vi "Evaluate Part 2.vi"() -> ()   [LabVIEW 2020]
uses:
  Stateless Network/Stateless Network.lvclass
panel:
  out "Steps":u64
  in  "Input":string
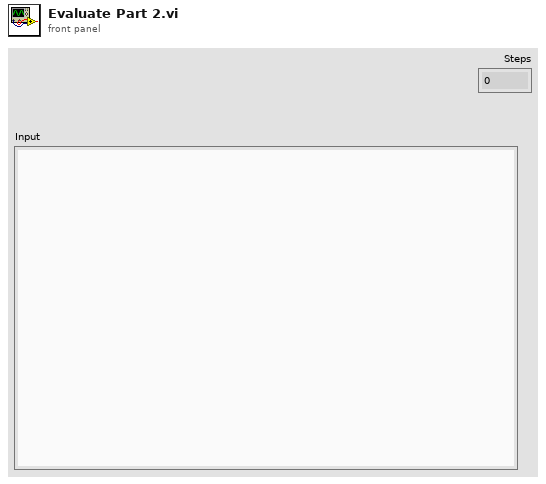
[diagram p1: front panel]
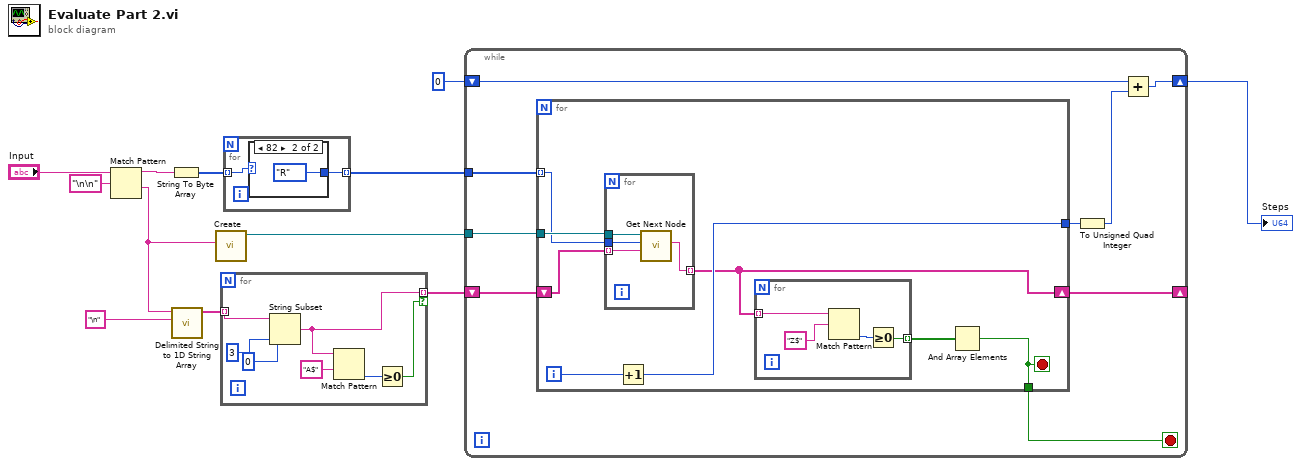
[diagram p0: block diagram]
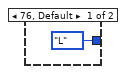
[diagram p2: hidden frame]
diagram:
  n1 = Match Pattern(string="Input", regular expression="\n\n" ("search string/char (-)")) -> (before substring=w10:string, after substring=w6:string)  [unwired: 1 in, 2 out]
  n2 = String To Byte Array(string=w10) -> (unsigned byte array=w9:u8[])
  n3 = call <vilib>:"Delimited String to 1D String Array.vi"("delimiter"="\n" ("search string/char (-)"), "delimited string"=w6) -> ("string array"=w2:string[])  [unwired: 9 in]
  n4 = call "Create.vi"("Input"=w6) -> ("Network"=w7:refnum<class "Stateless Network.lvclass">)  [unwired: 9 in, 1 out]
  n5 = for {
    tunnel: w2 -> [w14] mode=indexing
    tunnel: [w13] -> w1 mode=indexing if=w17
    n6 = String Subset(string=w14, offset (0)=0, length (rest)=3 ("length (rest)")) -> (substring=w13:string)
    n7 = Match Pattern(string=w13, regular expression="A$" ("y")) -> (offset past match=w18:i32)  [unwired: 1 in, 3 out]
    n8 = Greater Or Equal To 0?(x=w18) -> (x >= 0?=w17:bool)
  }
  n9 = for {
    tunnel: w9 -> [w21] mode=indexing
    tunnel: [w20] -> w8 mode=indexing
    n10 = case shown="82" w21 {
      tunnel: [enum16{"L", "R"}."L" ("Direction") enum16{"L", "R"}."R" ("Direction")] -> w20
      frame 76, Default {
      }
      frame 82 {
      }
    }
  }
  n11 = while {
    tunnel: w8 -> [w32]
    shift-right: [w27] -> _
    shift-left: w1 -> [w28]
    tunnel: w7 -> [w31]
    shift-right: [w25] -> w3
    shift-left: u64 0 -> [w26]
    stop <- w29 stop-if-true
    n12 = for {
      tunnel: w32 -> [w39] mode=indexing
      tunnel: [w37] -> w30
      tunnel: [w33] -> w29
      shift-right: [w35] -> w27
      shift-left: w28 -> [w36]
      tunnel: w31 -> [w40]
      i -> [w38]
      stop <- w33 stop-if-true
      n13 = for {
        tunnel: w39 -> [w47]
        tunnel: [w46] -> w35 mode=indexing
        tunnel: w36 -> [w45] mode=indexing
        tunnel: w40 -> [w48]
        n14 = call "Get Next Node.vi"("State"=w45, "Direction"=w47, "Network in"=w48) -> ("Node"=w46:string)  [unwired: 6 in, 2 out]
      }
      n15 = Increment(x=w38) -> (x+1=w37:i32)
      n16 = for {
        tunnel: w35 -> [w42] mode=indexing
        tunnel: [w41] -> w34 mode=indexing
        n17 = Match Pattern(string=w42, regular expression="Z$" ("y")) -> (offset past match=w43:i32)  [unwired: 1 in, 3 out]
        n18 = Greater Or Equal To 0?(x=w43) -> (x >= 0?=w41:bool)
      }
      n19 = And Array Elements(Boolean array=w34) -> (logical AND=w33:bool)
    }
    n20 = To Unsigned Quad Integer(1:w30) -> (0:w24:u64)
    n21 = Add(x=w26, y=w24) -> (x+y=w25:u64)
  }
  "Steps" <- w3
